vi "Get CITI Packages (All).vi"(8 "error in (no error)":errorcluster, 11 "CITI reference in":refnum<k24>) -> (0 "error out":errorcluster, 2 "CITI Packages":T1[](array[typedef]), 3 "CITI reference out":refnum<k24>)   [LabVIEW 2023, in "NI_HFNetworkAnalysis.lvlib"]
doc: "Retrieve all the CITI packages in memory for the referenced CITI file."
uses:
  NI_HFNetworkAnalysis.lvlib
  C:/srd-semi-rfcal-software/AuxTools/STSRFFixtureCharactUtility/Source/Code Modules/Fixture/Dependencies/HFNetworkAnalysis/Support Files/NACE.Utils.Data.dll
  Support Files/NACE.Utils.Data.dll
  Controls/CITI Package.ctl
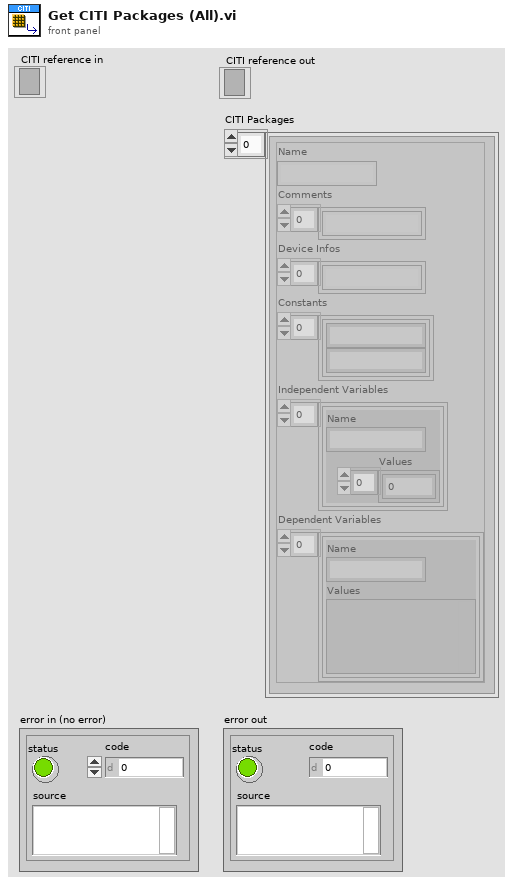
[diagram p1: front panel]
types:
  T1 = typedef "NI_HFNetworkAnalysis.lvlib/CITI Package.ctl" = cluster{"Name":string, "Comments":string[], "Device Infos":string[], "Constants":cluster{"Name":string, "Value":string}[], "Independent Variables":cluster{"Name":string, "Values":dbl[]}[], "Dependent Variables":cluster{"Name":string, "Values":variant}[]}
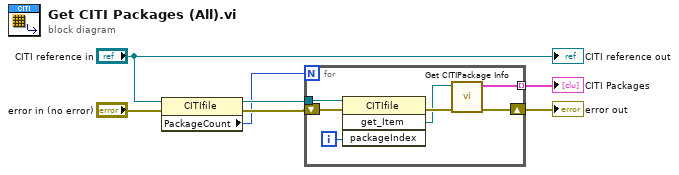
[diagram p0: block diagram]
diagram:
  n1 = property class="CITIfile"(reference="CITI reference in", error in="error in (no error)") -> (reference out=w5:refnum<k24>, error out=w6:errorcluster, "PackageCount"=w4:i32)
  n2 = for {
    N: w4 -> [_]
    tunnel: w5 -> [w14]
    tunnel: [w11] -> w2 mode=indexing
    shift-right: [w10] -> w3
    shift-left: w6 -> [w12]
    i -> [w13]
    n3 = invoke class="CITIfile" method="get_Item"(reference=w14, error in=w12, "packageIndex"=w13) -> (error out=w9:errorcluster, "get_Item"=w8:refnum<k24>)  [unwired: 1 in, 2 out]
    n4 = call "Get CITIPackage Info.vi"("error in (no error)"=w9, "CITI Package Refnum in"=w8) -> ("error out"=w10:errorcluster, "CITI Package"=w11:T1)  [unwired: 8 in]
  }
  "error out" <- w3
  "CITI Packages" <- w2
  "CITI reference out" <- "CITI reference in"
